vi "FTW-STR-Array-Delimit-Comma.vi"(5 "Array of Strings":string[](array[string])) -> (6 "Delimited String":string)   [LabVIEW 2015]
panel:
  # "Inputs"
  # "Outputs"
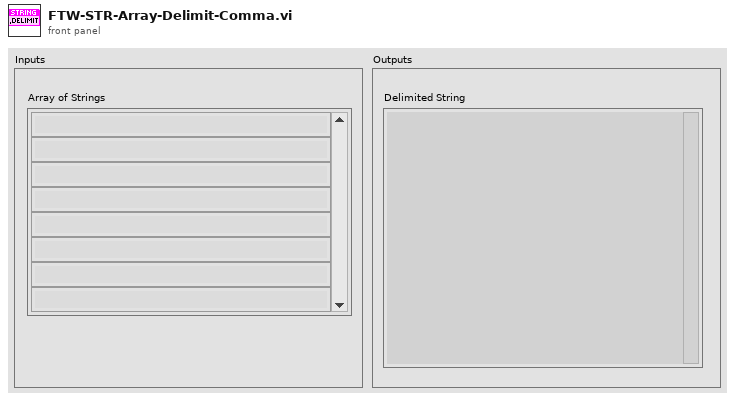
[diagram p1: front panel]
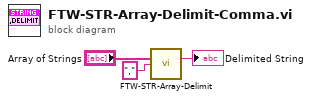
[diagram p0: block diagram]
diagram:
  n1 = call "FTW-STR-Array-Delimit.vi"("Array of Strings"="Array of Strings", "Delimiter"=",") -> ("Delimited String"=→"Delimited String":string)  [unwired: 13 in]
